vi "new FGGA Serial Data Server & Recordingv4.3_test.vi"(0 "VISA resource name out":refnum<visa-resource-name>, 11 "error IO":errorcluster) -> ()   [LabVIEW 2014]
uses:
  <vilib>/Platform/TimedLoop/XDataNode/timing_clust.ctl
  <vilib>/Platform/TimedLoop/XDataNode/nitl_modes.ctl
  <vilib>/Platform/TimedLoop/XDataNode/wakeup.ctl
  C:/Program Files (x86)/National Instruments/LabVIEW 2014/examples/Data Communication/Network Streams/Simple Network Streams/support/Network Stream Command.ctl
  <vilib>/Utility/error.llb/whitespace.ctl
  <vilib>/Instr/_visa.llb/VISA Flush IO Buffer Mask.ctl
  <vilib>/Instr/_visa.llb/VISA Configure Serial Port (Instr).vi
  <vilib>/Utility/tcp.llb/UDP Multicast Write-Only Open.vi
  <vilib>/platform/TimedLoop/XDataNode/XDataNode.xnode
  <vilib>/Platform/TimedLoop/XDataNode/XDNodeRunTimeDep.lvlib
panel:
  out "Waveform Chart":u32(graph)
  out "Max time diff":u32
  out "ASCII_file_out":string
  out "Unix time":u32
  out "FGGA Pump":bool
  out "Flight Number":string
  out "Stop File Write":bool
  out "Default file name":string
  out "MFC":dbl[](array[numeric])
  out "FGGA restart":bool
  out "V4":bool
  out "V3":bool
  out "V2":bool
  out "V1":bool
  out "error out 2":errorcluster
  out "error out":errorcluster
  in  "MFC_1 SLPM set value":dbl
  out "Value Read":string
  out "status":bool
  in  "VISA resource name":refnum<visa-resource-name>="ASRL3::INSTR"
  in  "timeout (10sec) 2":u32=3000
  in  "Clear Display\nErrors":bool
  out "Data Processing":bool
  out "TCP Binary Packet":string
  out "UDP Time Stamp Offset":i32=1
  out "Data String":string
  out "UDP_ACSII_Out":string
  out "Serial error out":errorcluster
  out "SEPTIC TCP Error Out":errorcluster
  out "TCP packet\nSend To SEPTIC":bool
  out "FISH TCP Error Out":errorcluster
  out "TCP packet\nSend To FISH":bool
  out "UDP_Pack_num":u32
  out "UDP_Out Status":bool
  out "UDP_Out_Error Out":errorcluster
  out "Data Array":string[](array[string])
  out "RAW DATA":string
  in  "stop":bool
  out "Number of times \nRead time out":u32
  out "Loop count":i32
  # "Date"
  # "Time"
  # "CH4_wet_ppm"
  # "1"
  # "CO4_wet_ppm_sd"
  # "H2O_ppm"
  # "3"
  # "H2O_ppm_sd"
  # "CO2_wet_ppm"
  # "5"
  # "CO2_wet_ppm_sd"
  # "CH4_dry_ppm"
  # "CH4_dry_ppm_sd"
  # "CO2_dry_ppm"
  # "CO2_dry_ppm_sd"
  # "cell_pressure_torr"
  # "11"
  # "cell_pressure_torr_sd"
  # "13"
  # "cell_temp_degC"
  # "cell_temp_degC_sdev"
  # "ambient(bench)_temp_degC"
  # "15"
  # "ambient(bench)_temp_dedgC_sd"
  # "17"
  # "RDA_us"
  # "RDA_us_sd"
  # "RDB_us"
  # "19"
  # "RDB_us_sd"
  # "Fitflag"
  # "21"
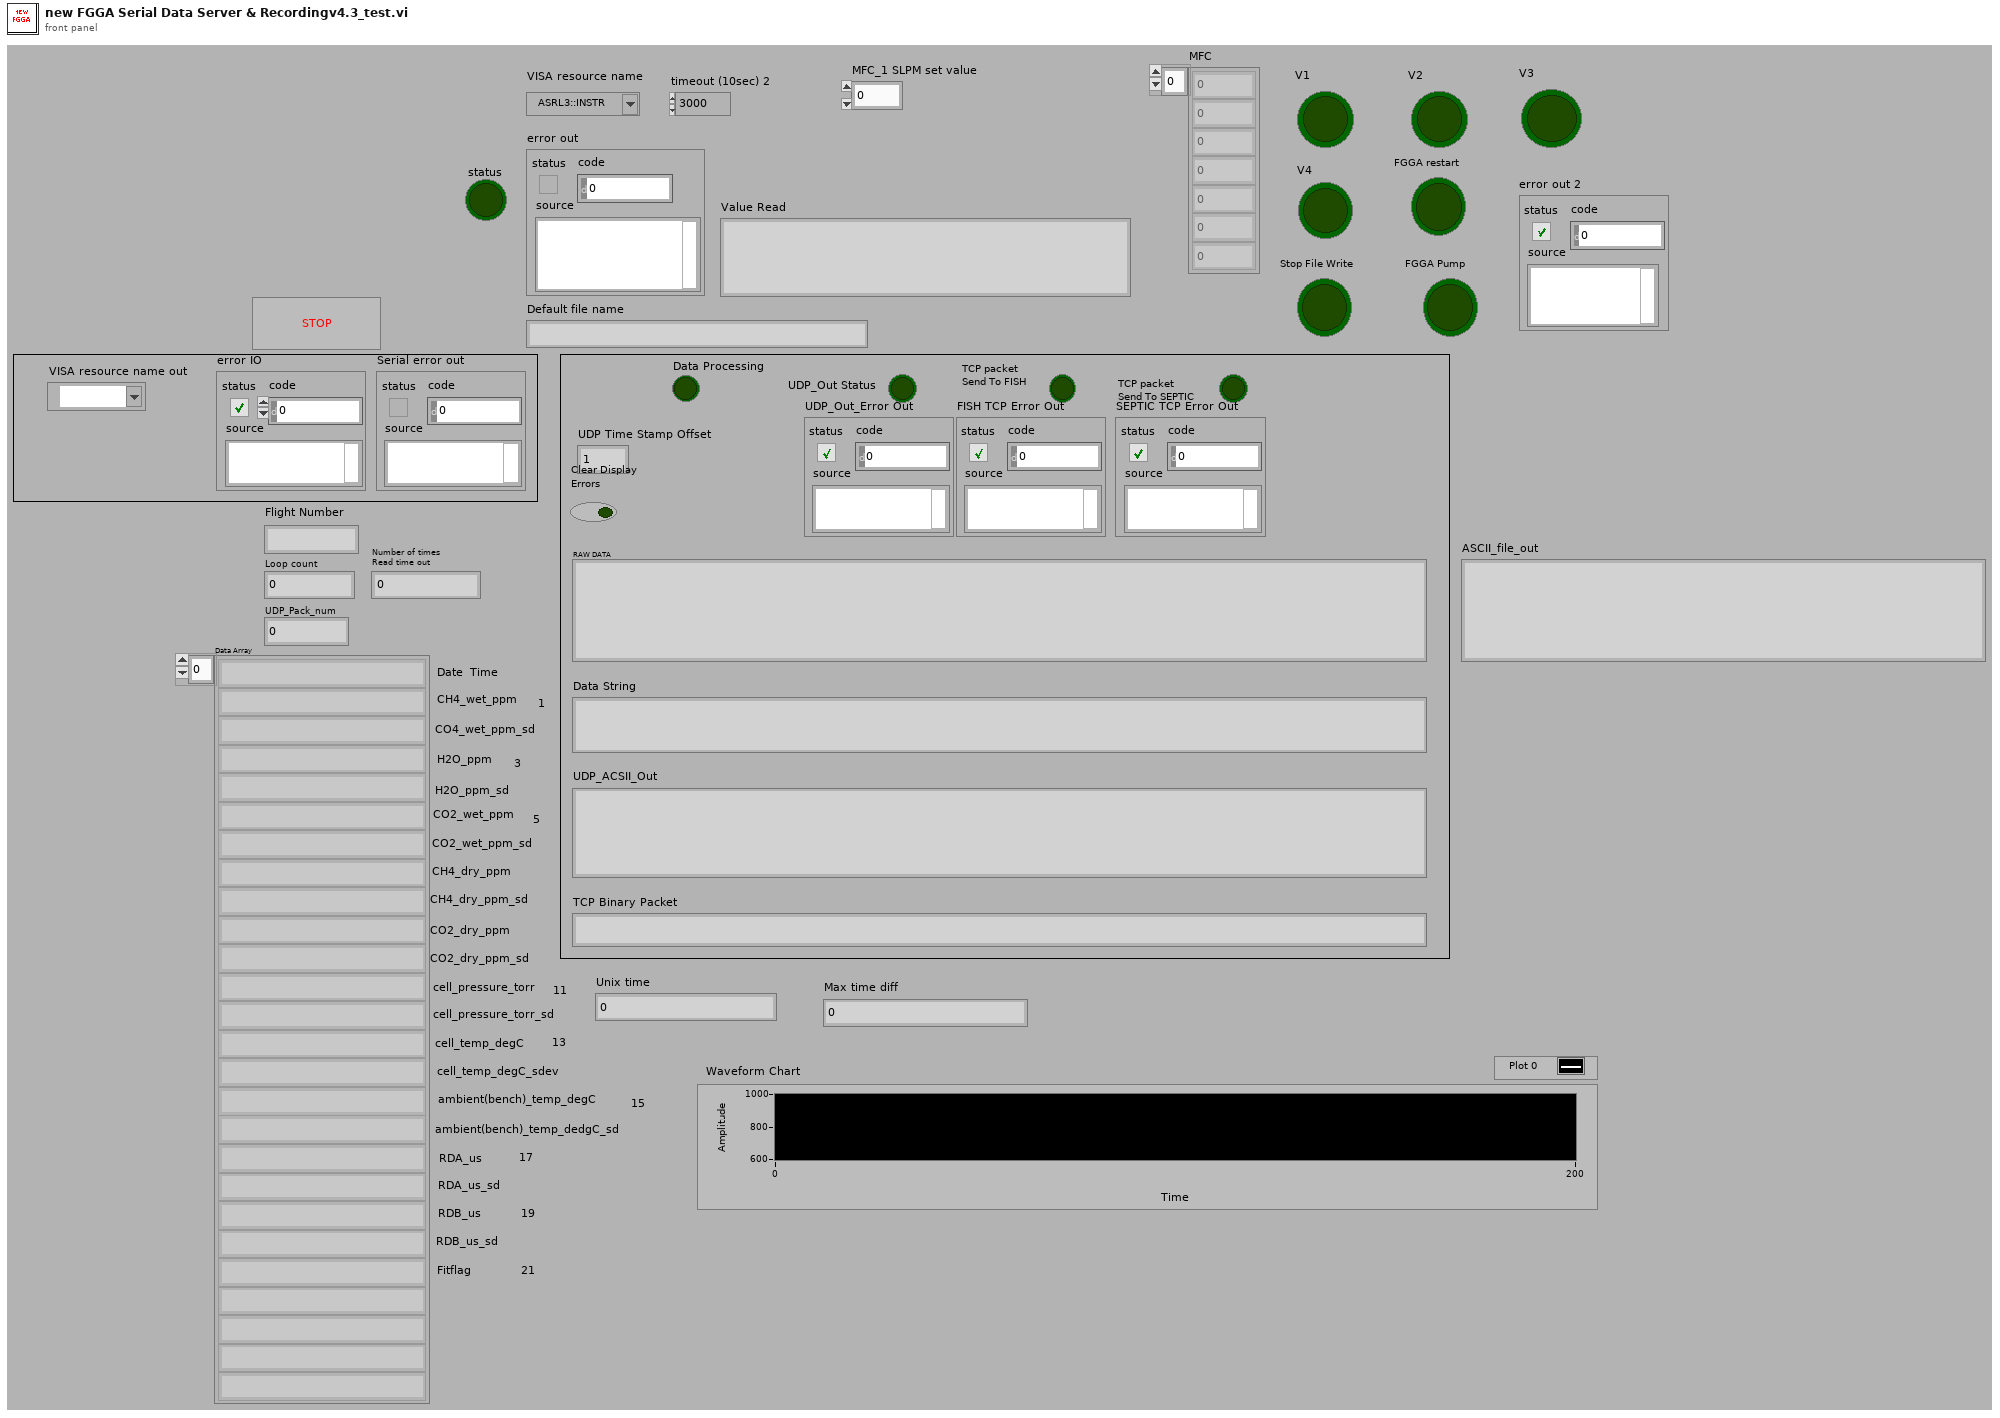
[diagram p1: front panel]
types:
  T1 = typedef "XDNodeRunTimeDep.lvlib/timing_clust.ctl" = cluster{"Expected End [f-1]":u64, "Actual End [f-1]":u64, "Finished Late? [f-1]":bool, "Expected End [i-1]":u64, "Actual End [i-1]":u64, "Finished Late? [i-1]":bool, "Expected Start [i]":u64, "Actual Start [i]":u64, "Expected Start [f]":u64, "Actual Start [f]":u64, "Source Name":string, "Structure Name":string, "Period":i64, "Deadline":i64, "Offset":i64, "Start":i64, "Priority":i32, "Timeout":i32, "Mode":T2, "Wakeup Reason":T3, "Error":errorcluster, "Source Type":string, "Secondary Source Type":string, "Global End Time":u64, "Global Start Time":u64, "Frame Duration":u64, "Iteration Duration":u64, "Assigned CPU":i32, "I/O Scan Engine Mode":u32}
  T2 = typedef "XDNodeRunTimeDep.lvlib/nitl_modes.ctl" = enum32{"No Change", "Process missed periods, maintain original phase", "Discard missed periods, maintain original phase", "Process missed periods, ignore original phase", "Discard missed periods, ignore original phase"}
  T3 = typedef "XDNodeRunTimeDep.lvlib/wakeup.ctl" = enum32{"Normal", "Aborted", "Asynchronous wakeup", "Timing source error", "Timed loop error", "Timeout"}
  T4 = enum16{"open", "replace", "create", "open or create", "replace or create", "replace or create with confirmation"}
  T5 = typedef "Network Stream Command.ctl" = cluster{"Message":string, "Message Data":variant}
  T6 = typedef "whitespace.ctl" = u16
  T7 = typedef "VISA Flush IO Buffer Mask.ctl" = u16
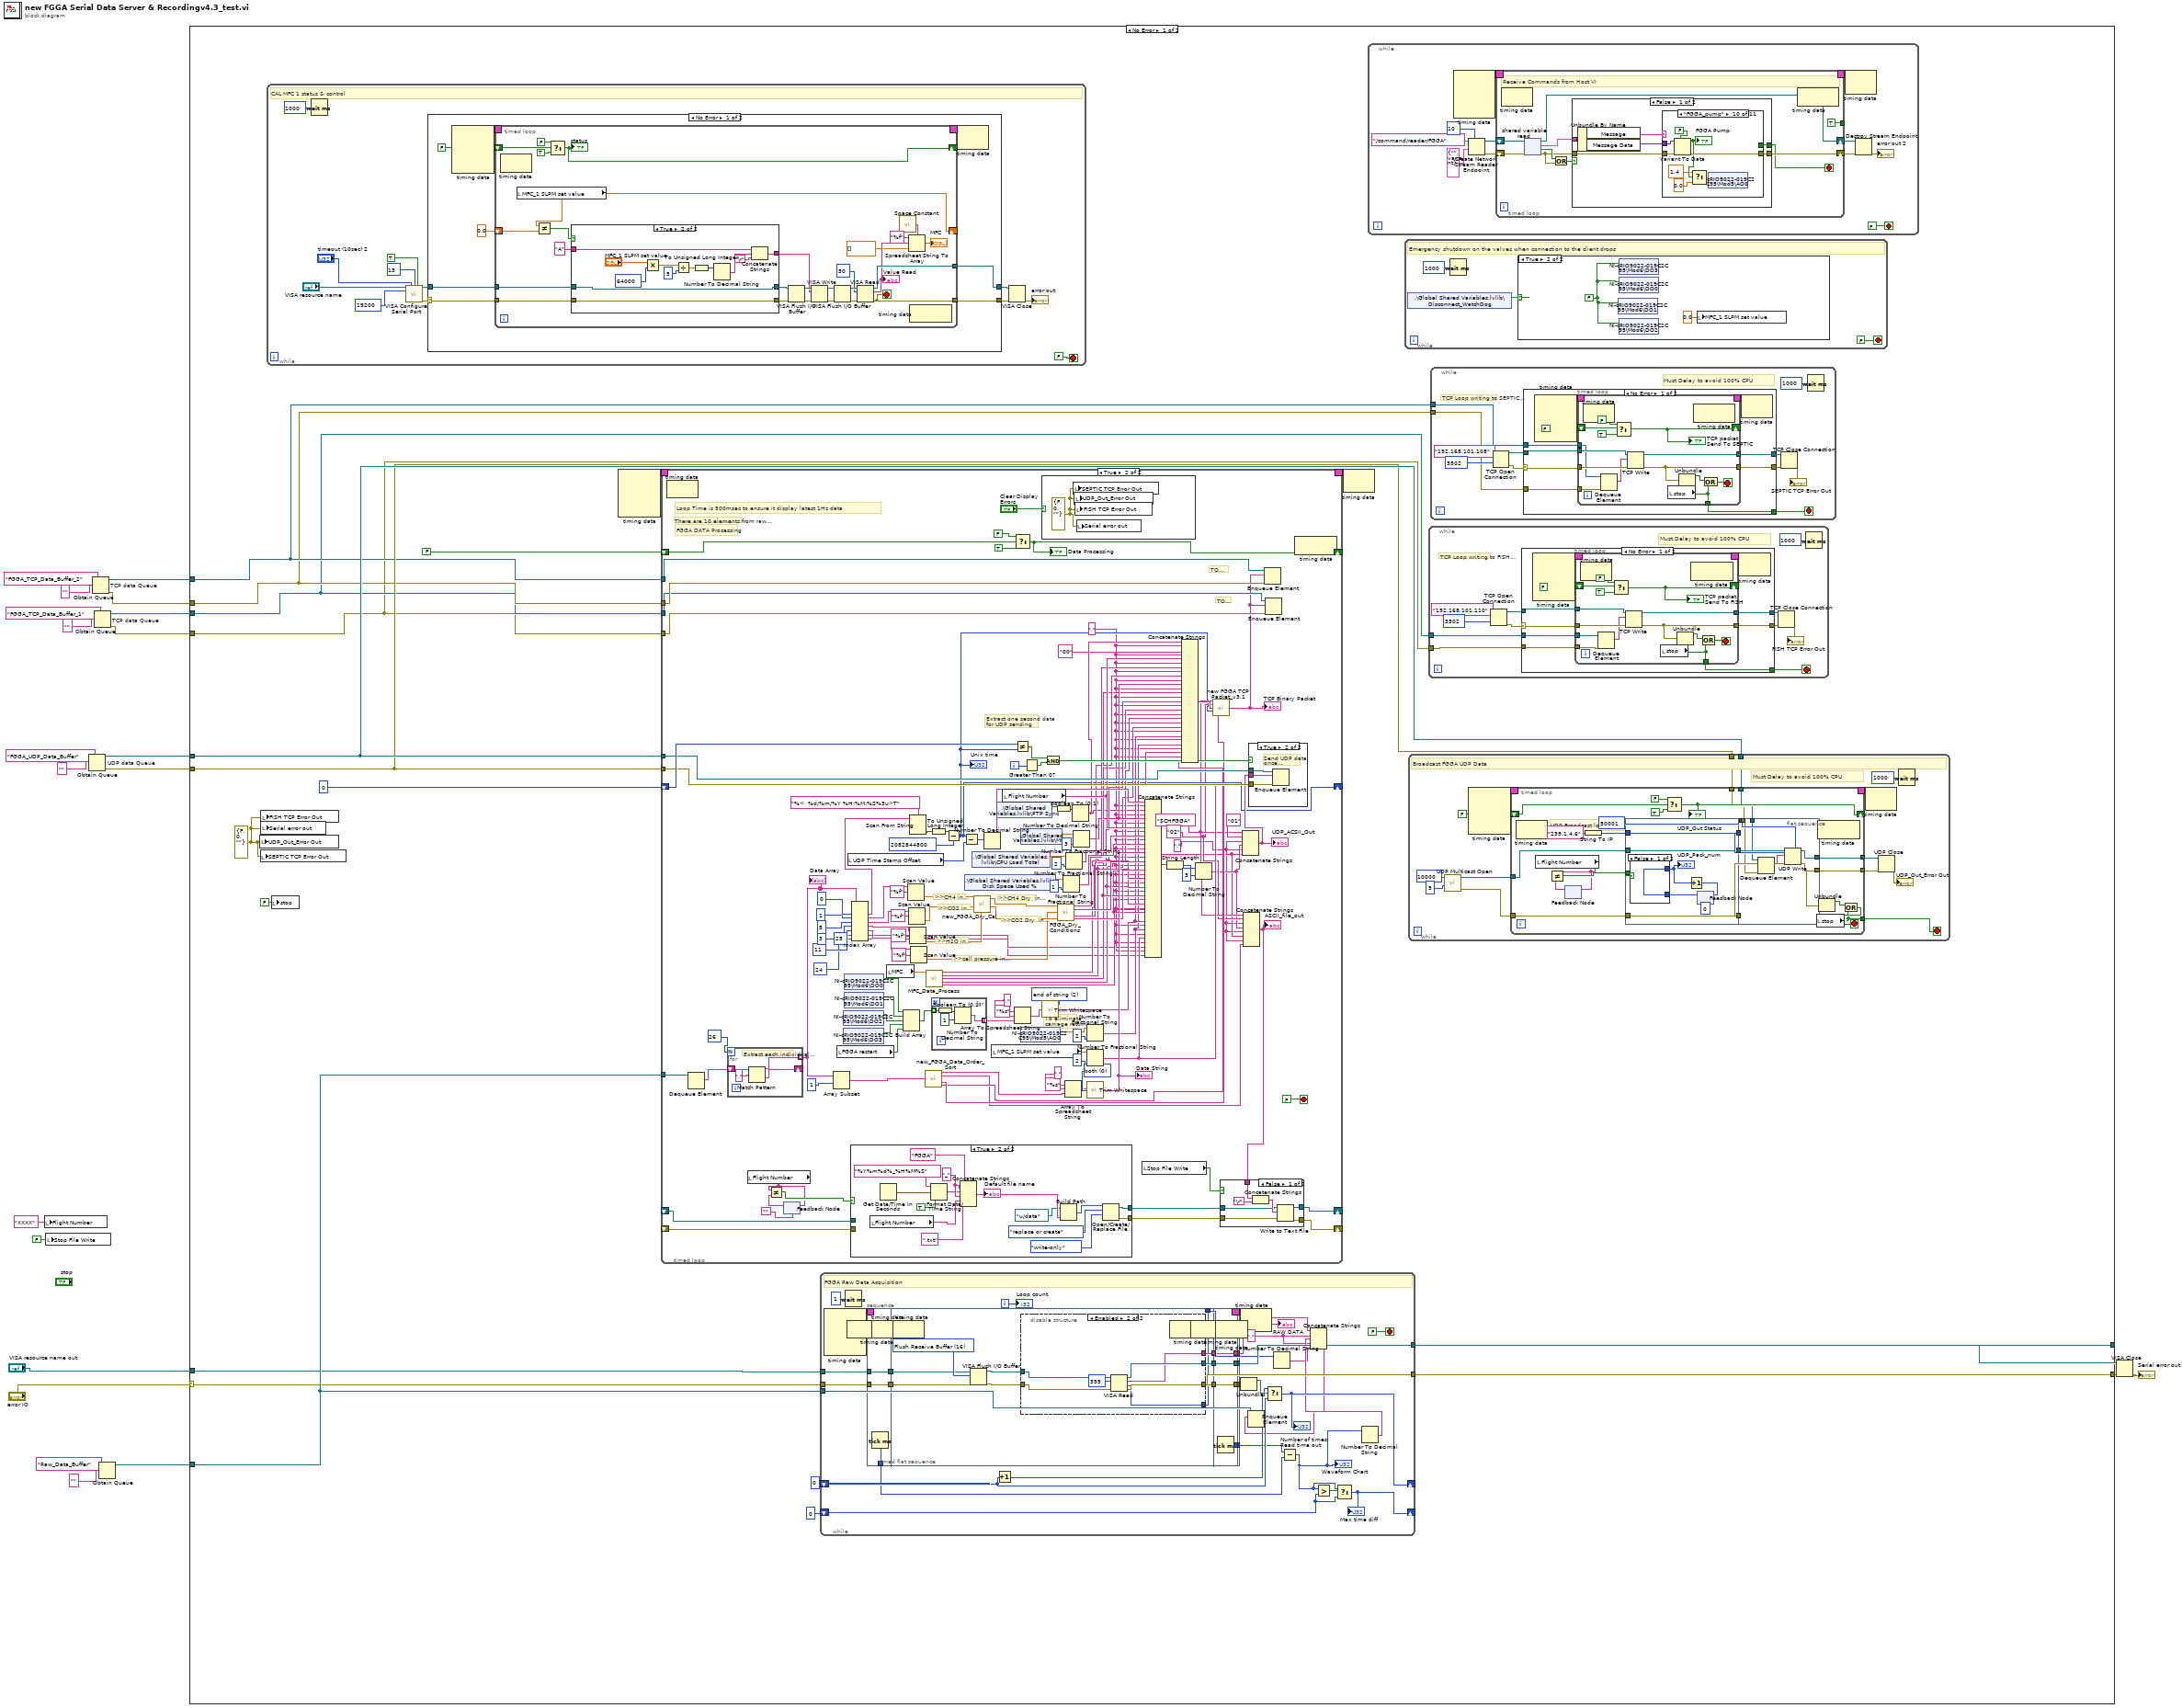
[diagram p0: block diagram]
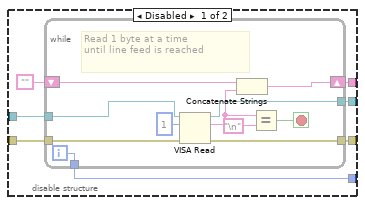
[diagram p2: hidden frame]
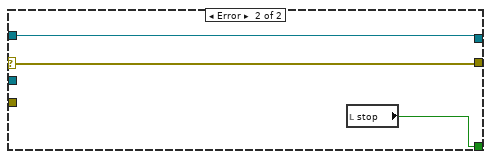
[diagram p3: hidden frame]
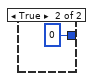
[diagram p4: hidden frame]
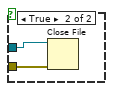
[diagram p6: hidden frame]
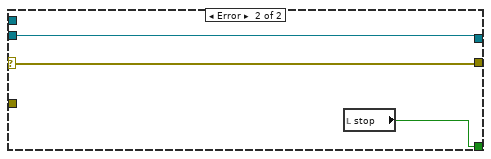
[diagram p9: hidden frame]
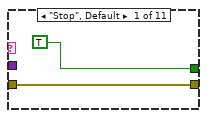
[diagram p11: hidden frame]
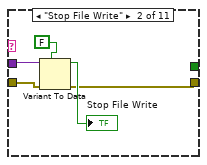
[diagram p12: hidden frame]
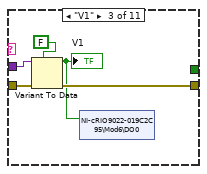
[diagram p13: hidden frame]
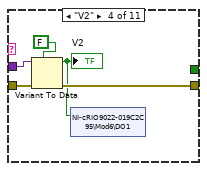
[diagram p14: hidden frame]
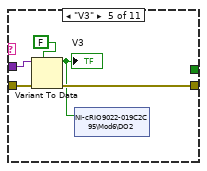
[diagram p15: hidden frame]
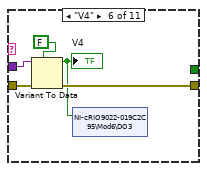
[diagram p16: hidden frame]
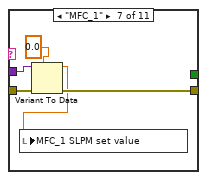
[diagram p17: hidden frame]
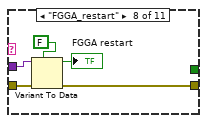
[diagram p18: hidden frame]
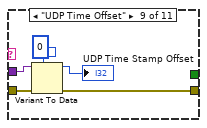
[diagram p19: hidden frame]
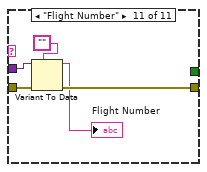
[diagram p20: hidden frame]
diagram:
  n1 = local write "Flight Number"("XXXX" ("Flight Number")) -> ()
  n2 = local write "Stop File Write"(FALSE ("Stop File Write")) -> ()
  n3 = Obtain Queue "UDP data Queue"(name (unnamed)="FGGA_UDP_Data_Buffer", element data type="") -> (queue out=w14:refnum<queue>, error out=w13:errorcluster)  [unwired: 3 in, 1 out]
  n4 = Obtain Queue "TCP data Queue"(name (unnamed)="FGGA_TCP_Data_Buffer_2", element data type="") -> (queue out=w8:refnum<queue>, error out=w7:errorcluster)  [unwired: 3 in, 1 out]
  n5 = Obtain Queue "TCP data Queue"(name (unnamed)="FGGA_TCP_Data_Buffer_1", element data type="") -> (queue out=w6:refnum<queue>, error out=w5:errorcluster)  [unwired: 3 in, 1 out]
  n6 = Obtain Queue(name (unnamed)="Raw_Data_Buffer", element data type="") -> (queue out=w20:refnum<queue>)  [unwired: 3 in, 2 out]
  n7 = case shown="No Error" "error IO" {
    selector: "error IO" -> [w28 w608]
    tunnel: "VISA resource name out" -> [w29 w609]
    tunnel: [w40 w609] -> w17
    tunnel: [w41 w608] -> w18
    tunnel: w20 -> [w39 _]
    tunnel: w14 -> [w37 _]
    tunnel: w13 -> [w36 _]
    tunnel: w8 -> [w35 _]
    tunnel: w7 -> [w34 _]
    tunnel: w6 -> [w33 _]
    tunnel: w5 -> [w32 _]
    frame No Error {
      w25 = errorcluster {"status"=FALSE, "code"=0, "source"=""} ("UDP Error Out")
      n8 = local write "UDP_Out_Error Out"(w25) -> ()
      n9 = local write "SEPTIC TCP Error Out"(w25) -> ()
      n10 = local write "FISH TCP Error Out"(w25) -> ()
      n11 = local write "Serial error out"(w25) -> ()
      n12 = while {
        stop <- FALSE stop-if-true
        # "CAL MFC 1 status & control"
        n13 = Wait (ms)(milliseconds to wait=u32 1000) -> ()  [unwired: 1 out]
        n14 = call-poly "VISA Configure Serial Port"("VISA resource name"="VISA resource name", "timeout (10sec)"="timeout (10sec) 2", "termination char\n(0xA = '\\n' = LF)"=u8 13 ("termination char\n(0xA = '\\n' = LF)"), "Enable Termination\nChar (T)"=TRUE ("Enable Termination\nChar (T)"), "baud rate (9600)"=u32 19200) -> ("VISA resource name out"=w549:refnum<visa-resource-name>, "error out"=w545:errorcluster)  [unwired: 9 in]
        n15 = case shown="No Error" w545 {
          selector: w545 -> [w556 w606]
          tunnel: w549 -> [w557 w607]
          tunnel: [w555 w607] -> w548
          tunnel: [w554 w606] -> w547
          frame No Error {
            n16 = node-c288() -> (w552:T1)  [unwired: 4 in]
            n17 = timed-loop {
              tunnel: w557 -> [w580]
              tunnel: w556 -> [w578]
              tunnel: [w571] -> w555
              tunnel: [w566] -> w554
              shift-right: [w567] -> _
              shift-left: FALSE -> [w570]
              timing: w552 -> [_]
              timing-out: [_] -> w551
              shift-right: [w558] -> _
              shift-left: 0.0 -> [w560]
              stop <- w566 stop-if-true
              n18 = node-c288() -> ()  [unwired: 1 in, 1 out]
              n19 = local read "MFC_1 SLPM set value"() -> (w558:dbl)
              n20 = Not Equal?(x=w558, y=w560) -> (x != y?=w559:bool)
              n21 = Select(t=FALSE, s=w570, f=TRUE) -> (s? t:f=w567:bool)
              "status" <- w567
              n22 = case shown="True" w559 {
                tunnel: w580 -> [w588 w603]
                tunnel: [w588 w603] -> w579
                tunnel: w578 -> [w587 w602]
                tunnel: [w587 w602] -> w577
                tunnel: "A" -> [w591 w595]
                tunnel: [w589 w592] -> w575
                frame False {
                  n23 = Concatenate Strings(w591, "\r") -> (w589:string)
                }
                frame True {
                  n24 = Multiply(x="MFC_1 SLPM set value", y=u32 64000) -> (x*y=w599:dbl)
                  n25 = Divide(x=w599, y=u32 5) -> (x/y=w597:dbl)
                  n26 = To Unsigned Long Integer(number=w597) -> (unsigned 32bit integer=w596:u32)
                  n27 = Number To Decimal String(number=w596) -> (decimal integer string=w594:string)  [unwired: 1 in]
                  n28 = Concatenate Strings(w595, w594, "\r") -> (w592:string)
                }
              }
              n29 = VISA Flush I/O Buffer(VISA resource name=w579, error in (no error)=w577) -> (VISA resource name out=w582:refnum<visa-resource-name>, error out=w581:errorcluster)  [unwired: 1 in]
              n30 = VISA Write(VISA resource name=w582, write buffer=w575, error in (no error)=w581) -> (VISA resource name out=w574:refnum<visa-resource-name>, error out=w573:errorcluster)  [unwired: 1 out]
              n31 = VISA Flush I/O Buffer(VISA resource name=w574, error in (no error)=w573) -> (VISA resource name out=w584:refnum<visa-resource-name>, error out=w583:errorcluster)  [unwired: 1 in]
              n32 = VISA Read(VISA resource name=w584, byte count=u32 50, error in (no error)=w583) -> (VISA resource name out=w571:refnum<visa-resource-name>, read buffer=w565:string, error out=w566:errorcluster)  [unwired: 1 out]
              "Value Read" <- w565
              n33 = call <vilib>:"Space Constant.vi"() -> ("String"=w564:string)
              n34 = Spreadsheet String To Array(delimiter (Tab)=w564, format string="%f", spreadsheet string=w565, array type (2D Dbl)=dbl[] []) -> (array=→"MFC":dbl[])
              n35 = node-c288() -> ()  [unwired: 1 in, 1 out]
            }
            n36 = node-c288(w551) -> ()  [unwired: 1 out]
          }
          frame Error {
          }
        }
        n37 = VISA Close(VISA resource name=w548, error in (no error)=w547) -> (error out=→"error out":errorcluster)
      }
      n38 = local write "stop"(FALSE ("stop")) -> ()
      n39 = node-c288() -> (w27:T1)  [unwired: 4 in]
      n40 = timed-loop {
        timing: w27 -> [_]
        timing-out: [_] -> w26
        tunnel: w39 -> [w360]
        tunnel: w37 -> [w328]
        tunnel: w36 -> [w327]
        shift-right: [w255] -> _
        shift-left: u32 0 -> [w331]
        tunnel: w35 -> [w326]
        tunnel: w34 -> [w325]
        tunnel: w33 -> [w324]
        tunnel: w32 -> [w323]
        shift-right: [w319] -> _
        shift-left: FALSE -> [w322]
        shift-right: [w308] -> _
        shift-left: _ -> [w300]
        shift-right: [w298] -> _
        shift-left: _ -> [w299]
        i -> [w330]
        stop <- FALSE stop-if-true
        w272 = T6 2 items=["both", "start of string", "end of string"] ("location (both)")
        w233 = ","
        w349 = T6 0 items=["both", "start of string", "end of string"] ("location (both)")
        w237 = ","
        w241 = "02"
        w242 = "$CHFGGA"
        # "To eliminate\ncarriage return"
        # ">>cell pressure in torr>>"
        # "There are 10 elements from raw packet"
        # "TO SEPTIC"
        # "TO FISH"
        # "Extract one second data\nfor UDP sending"
        # ">>CO2 Dry  in ppm>>"
        # ">>CH4 Dry  in ppb>>"
        # ">>H2O in ppm>>"
        # ">>CO2 in ppm>>"
        # ">>CH4 in ppm>>"
        # "Loop Time is 500msec to ensure it display latest 1Hz data"
        # "FGGA DATA Processing"
        n41 = node-c288() -> ()  [unwired: 1 in, 1 out]
        n42 = Dequeue Element(queue=w360) -> (element=w318:string)  [unwired: 2 in, 3 out]
        n43 = for {
          N: 26 -> [_]
          shift-right: [w397] -> _
          shift-left: w318 -> [w395]
          tunnel: [w396] -> w354 mode=indexing
          # "Extract each individual param"
          n44 = Match Pattern(string=w395, regular expression=",") -> (before substring=w396:string, after substring=w397:string)  [unwired: 1 in, 2 out]
        }
        "Data Array" <- w354
        n45 = local read "Flight Number"() -> (w297:string)
        n46 = feedback #1("" ("Flight Number")) -> (w305:string)
        n47 = Not Equal?(x=w297, y=w305) -> (x != y?=w303:bool)
        n48 = feedback-in #1(w297) -> ()
        n49 = Array Subset(array=w354, index=1) -> (w247:string[])  [unwired: 1 in]
        n50 = local read "FGGA restart"() -> (w282:bool)
        n51 = shared-variable "NI-cRIO9022-019C2C95\\Mod6\\DO2"() -> (w288:bool)  [unwired: 1 in, 1 out]
        n52 = shared-variable "NI-cRIO9022-019C2C95\\Mod6\\DO3"() -> (w287:bool)  [unwired: 1 in, 1 out]
        n53 = shared-variable "NI-cRIO9022-019C2C95\\Mod6\\DO0"() -> (w290:bool)  [unwired: 1 in, 1 out]
        n54 = shared-variable "NI-cRIO9022-019C2C95\\Mod6\\DO1"() -> (w289:bool)  [unwired: 1 in, 1 out]
        n55 = local read "UDP Time Stamp Offset"() -> (w271:i32)
        n56 = case shown="True" w303 {
          tunnel: [w366 w368] -> w302
          tunnel: [w365 w367] -> w301
          tunnel: w300 -> [w366 _]
          tunnel: w299 -> [w365 _]
          frame False {
          }
          frame True {
            w374 = "_" ("string")
            n57 = local read "Flight Number"() -> (w381:string)
            n58 = Get Date/Time In Seconds() -> (seconds since 1Jan1904=w369:timestamp)
            n59 = Format Date/Time String(time format string (%c)="%Y%m%d%_%H%M%S", seconds (now)=w369, UTC format=TRUE) -> (date/time string=w371:string)
            n60 = Concatenate Strings("FGGA" ("string"), w374, w371, w374, w381, ".txt" ("string")) -> (w376:string)
            "Default file name" <- w376
            n61 = Build Path(base path=path "u:/data", name or relative path=w376) -> (appended path=w380:path)
            n62 = Open/Create/Replace File(file path (use dialog)=w380, operation (0:open)=T4."replace or create", access (0:read/write)=enum16{"read/write", "read-only", "write-only"}."write-only") -> (refnum out=w368:refnum<file>, error out=w367:errorcluster)  [unwired: 3 in, 1 out]
          }
        }
        n63 = Index Array(array=w354, index #1=0 ("index"), index #2=1 ("index"), index #3=5 ("index"), index #4=3 ("index"), index #5=11 ("index"), index #6=24 ("index"), index #7=25 ("index")) -> (element #1=w249:string, element #2=w254:string, element #3=w253:string, element #4=w252:string, element #5=w251:string, element #6=w234:string, element #7=w231:string)
        n64 = local read "MFC"() -> (w309:dbl[])
        n65 = Build Array(w290, w289, w288, w287, w282) -> (w286:bool[])
        n66 = Scan Value(string=w254, format string="%f") -> (value=w340:dbl)  [unwired: 1 in, 1 out]
        n67 = Scan Value(string=w253, format string="%f") -> (value=w339:dbl)  [unwired: 1 in, 1 out]
        n68 = Scan From String(format string="%<  %d/%m/%Y %H:%M:%S%3u>T", input string=w249) -> (output 1=w336:timestamp)  [unwired: 3 in, 3 out]
        n69 = Scan Value(string=w252, format string="%f") -> (value=w310:dbl)  [unwired: 1 in, 1 out]
        n70 = Scan Value(string=w251, format string="%f") -> (value=w311:dbl)  [unwired: 1 in, 1 out]
        n71 = call "new_FGGA_Data_Order_Sort.vi"("Data In"=w247) -> ("UDP Data Out"=w246:string[], "ASCII Ambient(bench)_temp"=w236:string, "TCP Data Out"=w245:string[], "TCP Ambient(bench)_temp"=w244:string)  [unwired: 11 in]
        n72 = call "MFC_Data_Process.vi"("MFC"=w309) -> ("MFC Absolute Pressure"=w266:string, "MFC Temperature"=w265:string, "MFC Volumetric Flow"=w264:string, "MFC Mass Flow"=w263:string, "MFC Set Point"=w262:string)  [unwired: 10 in]
        n73 = To Unsigned Long Integer(number=w336) -> (unsigned 32bit integer=w337:u32)
        n74 = for {
          tunnel: w286 -> [w363] mode=indexing
          tunnel: [w362] -> w283 mode=indexing
          n75 = Boolean To (0,1)(Boolean=w363) -> (0, 1=w364:i16)
          n76 = Number To Decimal String(number=w364, width (-)=i16 1) -> (decimal integer string=w362:string)
        }
        n77 = Subtract(x=w337, y=u32 2082844800) -> (x-y=w255:u32)
        "Unix time" <- w255
        n78 = Subtract(x=w255, y=w271) -> (x-y=w334:u32)
        n79 = shared-variable ".\\Global Shared Variables.lvlib\\Disk Space Used %"() -> (w275:dbl)  [unwired: 1 in, 1 out]
        n80 = shared-variable ".\\Global Shared Variables.lvlib\\CPU Load Total"() -> (w296:dbl)  [unwired: 1 in, 1 out]
        n81 = call "new_FGGA_Dry_Cal.vi"("H2O"=w310, "CO2_Wet"=w339, "CH4_Wet"=w340) -> ("CO2_Dry"=w313:dbl, "CH4_Dry"=w315:dbl)  [unwired: 7 in]
        n82 = Number To Decimal String(number=w334) -> (decimal integer string=w335:string)  [unwired: 1 in]
        n83 = local read "MFC_1 SLPM set value"() -> (w278:dbl)
        n84 = shared-variable ".\\Global Shared Variables.lvlib\\PTP Sync"() -> (w291:bool)  [unwired: 1 in, 1 out]
        n85 = local read "Flight Number"() -> (w270:string)
        n86 = Array To Spreadsheet String(delimiter (Tab)=",", array=w283, 3:"%s" ("format string")) -> (spreadsheet string=w273:string)
        n87 = Select(t=FALSE, s=w322, f=TRUE) -> (s? t:f=w319:bool)
        "Data Processing" <- w319
        n88 = Not Equal?(x=w331, y=w255) -> (x != y?=w332:bool)
        n89 = shared-variable ".\\Global Shared Variables.lvlib\\MFM"() -> (w294:dbl)  [unwired: 1 in, 1 out]
        n90 = shared-variable "NI-cRIO9022-019C2C95\\Mod5\\AO0"() -> (w280:dbl)  [unwired: 1 in, 1 out]
        n91 = Greater Than 0?(x=w330) -> (x > 0?=w333:bool)
        n92 = case shown="True" "Clear Display\nErrors" {
          frame False {
          }
          frame True {
            w391 = errorcluster {"status"=FALSE, "code"=0, "source"=""} ("UDP Error Out")
            n93 = local write "SEPTIC TCP Error Out"(w391) -> ()
            n94 = local write "UDP_Out_Error Out"(w391) -> ()
            n95 = local write "FISH TCP Error Out"(w391) -> ()
            n96 = local write "Serial error out"(w391) -> ()
          }
        }
        n97 = call <vilib>:"Trim Whitespace.vi"("string"=w273, "location (both)"=w272) -> ("trimmed string"=w261:string)
        n98 = Compound Arithmetic op=AND(w332, w333) -> (w329:bool)
        n99 = Boolean To (0,1)(Boolean=w291) -> (0, 1=w292:i16)
        n100 = call "FGGA_Dry_Conditions.vi"("CH4_Dry"=w315, "Pressure"=w311, "CO2_Dry"=w313) -> ("CH4_Dry_TCP"=w269:string, "CH4_Dry_UDP"=w317:string, "CO2_Dry_TCP"=w268:string, "CO2_Dry_UDP"=w316:string)  [unwired: 9 in]
        n101 = Number To Fractional String(number=w275, precision (6)=i16 1) -> (F-format string=w274:string)  [unwired: 2 in]
        n102 = Array To Spreadsheet String(delimiter (Tab)=",", array=w246, 3:"%s" ("format string")) -> (spreadsheet string=w348:string)
        n103 = Number To Fractional String(number=w296, precision (6)=i16 2) -> (F-format string=w277:string)  [unwired: 2 in]
        n104 = Number To Decimal String(number=w292) -> (decimal integer string=w257:string)  [unwired: 1 in]
        n105 = Number To Fractional String(number=w294, precision (6)=i16 3) -> (F-format string=w267:string)  [unwired: 2 in]
        n106 = Number To Fractional String(number=w280, precision (6)=i16 2) -> (F-format string=w260:string)  [unwired: 2 in]
        n107 = Number To Fractional String(number=w278, precision (6)=i16 2) -> (F-format string=w259:string)  [unwired: 2 in]
        n108 = call <vilib>:"Trim Whitespace.vi"("string"=w348, "location (both)"=w349) -> ("trimmed string"=w347:string)
        "Data String" <- w347
        n109 = local read "Stop File Write"() -> (w306:bool)
        n110 = Concatenate Strings(w335, w233, w257, w233, w267, w233, w270, w233, w277, w233, w274, w233, w347, w233, w317, w233, w316, w233, w266, w233, w265, w233, w264, w233, w263, w233, w262, w233, w261, w233, w260, w233, w259, w233, w234, w233, w231) -> (w239:string)
        n111 = String Length(string=w239) -> (length=w357:i32)
        n112 = Concatenate Strings(w257, w233, "00", w233, w270, w233, w269, w233, w268, w233, w267, w233, w266, w233, w265, w233, w264, w233, w263, w233, w262, w233, w261, w233, w260, w233, w259, w233, w244) -> (w258:string)
        n113 = Number To Decimal String(number=w357, width (-)=i16 3) -> (decimal integer string=w240:string)
        n114 = call "new FGGA TCP Packet_v3.1.vi"("ID"=w242, "Version"=w241, "TCP Packet In"=w258, "utc_time"=w255, "Data Array"=w245) -> ("TCP Binary Packet"=w248:string)  [unwired: 10 in]
        "TCP Binary Packet" <- w248
        n115 = Concatenate Strings(w242, "01", w237, w240, w237, w239) -> (w307:string)
        "UDP_ACSII_Out" <- w307
        n116 = Concatenate Strings(w242, w241, w237, w240, w237, w239, w237, w236) -> (w238:string)
        "ASCII_file_out" <- w238
        n117 = case shown="False" w306 {
          tunnel: w238 -> [w388 _]
          tunnel: [w385 _] -> w308
          tunnel: w302 -> [w384 w390]
          tunnel: w301 -> [w383 w389]
          tunnel: [w382 _] -> w298
          frame False {
            n118 = Concatenate Strings(w388, "\r") -> (w386:string)
            n119 = Write to Text File(file (use dialog)=w384, text=w386, error in=w383) -> (refnum out=w385:refnum<file>, error out=w382:errorcluster)  [unwired: 2 out]
          }
          frame True {
            n120 = Close File(refnum=w390, error in=w389) -> ()  [unwired: 2 out]
          }
        }
        n121 = case shown="True" w329 {
          tunnel: w307 -> [_ w394]
          tunnel: w328 -> [_ w393]
          tunnel: w327 -> [_ w392]
          frame False {
          }
          frame True {
            # "Send UDP data once\na second"
            n122 = Enqueue Element(queue=w393, element=w394, error in (no error)=w392) -> ()  [unwired: 1 in, 3 out]
          }
        }
        n123 = Enqueue Element(queue=w326, element=w248, error in (no error)=w325) -> ()  [unwired: 1 in, 3 out]
        n124 = Enqueue Element(queue=w324, element=w248, error in (no error)=w323) -> ()  [unwired: 1 in, 3 out]
        n125 = node-c288() -> ()  [unwired: 1 in, 1 out]
      }
      n126 = while {
        tunnel: w29 -> [w57]
        tunnel: w28 -> [w56]
        tunnel: [w67] -> w41
        shift-right: [w63] -> _
        shift-left: u32 0 -> [w64]
        tunnel: [w66] -> w40
        tunnel: w39 -> [w61]
        shift-right: [w51] -> _
        shift-left: u32 0 -> [w52]
        i -> [w65]
        stop <- FALSE stop-if-true
        w45 = ","
        # "FGGA Raw Data Acquisition"
        n127 = node-c288() -> (w43:T1)  [unwired: 4 in]
        n128 = Wait (ms)(milliseconds to wait=u32 1) -> ()  [unwired: 1 out]
        n129 = timed-sequence {
          timing: w43 -> [_]
          timing-out: [_] -> w42
          tunnel: w57 -> [w80]
          tunnel: w56 -> [w79]
          tunnel: [w78] -> w54
          tunnel: [w75] -> w46
          tunnel: [w73] -> w67
          tunnel: [w71] -> w66
          tunnel: [w69] -> w49
          tunnel: [w68] -> w55
          n130 = timed-flat-sequence {
            tunnel: w79 -> [w82]
            tunnel: w80 -> [w83]
            tunnel: [w83] -> w77
            tunnel: [w82] -> w76
            tunnel: [w81] -> w78
            tunnel: w77 -> [w88]
            tunnel: w76 -> [w87]
            tunnel: [w94] -> w74
            tunnel: [w93] -> w72
            tunnel: [w92] -> w70
            tunnel: [w86] -> w75
            tunnel: [w123] -> w69
            tunnel: [w124] -> w71
            tunnel: [w125] -> w73
            tunnel: w74 -> [w125]
            tunnel: w72 -> [w124]
            tunnel: w70 -> [w123]
            tunnel: [w122] -> w68
            frame #0 {
              n131 = node-c288() -> ()  [unwired: 1 in, 1 out]
              n132 = node-c288() -> ()  [unwired: 1 in, 1 out]
              n133 = Tick Count (ms)() -> (millisecond timer value=w81:u32)
            }
            frame #1 {
              w89 = T7 16 items=["Flush Receive Buffer"=16, "Write Transmit Buffer to Device"=32, "Flush Receive Buffer (No I/O)"=64, "Flush Transmit Buffer"=128] ("Mask")
              n134 = node-c288() -> ()  [unwired: 1 in, 1 out]
              n135 = VISA Flush I/O Buffer(VISA resource name=w88, mask (16)=w89, error in (no error)=w87) -> (VISA resource name out=w90:refnum<visa-resource-name>, error out=w91:errorcluster)
              n136 = disable-structure shown="Enabled" {
                disable-tunnel: [w103 w119] -> w94
                disable-tunnel: [w102 w118] -> w93
                disable-tunnel: [w101 w117] -> w92
                disable-tunnel: w91 -> [w100 w120]
                disable-tunnel: w90 -> [w99 w121]
                disable-tunnel: [w97 w115] -> w86
                frame Disabled {
                  n137 = while {
                    tunnel: [w114] -> w102
                    tunnel: [w113] -> w103
                    tunnel: w99 -> [w112]
                    tunnel: w100 -> [w111]
                    shift-right: [w109] -> w101
                    shift-left: "" -> [w110]
                    tunnel: [w104] -> w97
                    i -> [w104]
                    stop <- w106 stop-if-true
                    # "Read 1 byte at a time \nuntil line feed is reached"
                    n138 = VISA Read(VISA resource name=w112, byte count=u32 1, error in (no error)=w111) -> (VISA resource name out=w114:refnum<visa-resource-name>, read buffer=w108:string, error out=w113:errorcluster)  [unwired: 1 out]
                    n139 = Concatenate Strings(w110, w108) -> (w109:string)
                    n140 = Equal?(x=w108, y="\n") -> (x = y?=w106:bool)
                  }
                }
                frame Enabled {
                  n141 = VISA Read(VISA resource name=w121, byte count=u32 395, error in (no error)=w120) -> (VISA resource name out=w118:refnum<visa-resource-name>, read buffer=w117:string, return count=w115:u32, error out=w119:errorcluster)
                }
              }
              n142 = node-c288() -> ()  [unwired: 1 in, 1 out]
            }
            frame #2 {
              n143 = node-c288() -> ()  [unwired: 1 in, 1 out]
              n144 = node-c288() -> ()  [unwired: 1 in, 1 out]
              n145 = Tick Count (ms)() -> (millisecond timer value=w122:u32)
            }
          }
        }
        "RAW DATA" <- w49
        n146 = Increment(x=w64) -> (x+1=w62:u32)
        n147 = node-c288(w42) -> ()  [unwired: 1 out]
        n148 = Unbundle(w67) -> ("status"=w60:bool)  [unwired: 2 out]
        n149 = Select(t=w62, s=w60, f=w64) -> (s? t:f=w63:u32)
        "Number of times \nRead time out" <- w63
        n150 = Number To Decimal String(number=w46) -> (decimal integer string=w44:string)  [unwired: 1 in]
        n151 = Subtract(x=w55, y=w54) -> (x-y=w50:u32)
        "Waveform Chart" <- w50
        n152 = Greater?(x=w50, y=w52) -> (0:w53:bool)
        n153 = Select(t=w50, s=w53, f=w52) -> (s? t:f=w51:u32)
        "Max time diff" <- w51
        n154 = Number To Decimal String(number=w50) -> (decimal integer string=w48:string)  [unwired: 1 in]
        n155 = Concatenate Strings(w49, w45, w48, w45, w44) -> (w47:string)
        n156 = Enqueue Element(queue=w61, element=w47) -> ()  [unwired: 2 in, 3 out]
        "Loop count" <- w65
      }
      n157 = node-c288(w26) -> ()  [unwired: 1 out]
      n158 = while {
        stop <- FALSE stop-if-true
        n159 = node-c288() -> (w451:T1)  [unwired: 4 in]
        n160 = Create Network Stream Reader Endpoint(7:10 ("reader buffer size"), 9:T5 {"Message"="", "Message Data"=variant} ("Message Cluster"), 11:"/command/reader/FGGA" ("reader url")) -> (0:w456:errorcluster, 3:w457:refnum<k21>)  [unwired: 4 in]
        n161 = timed-loop "Host->Target Command Reader" {
          shift-right: [w467] -> w454
          shift-left: w456 -> [w470]
          shift-right: [w468] -> w453
          shift-left: w457 -> [w469]
          tunnel: [TRUE] -> _
          timing: w451 -> [_]
          timing-out: [_] -> w450
          stop <- w461 stop-if-true
          # "Receive Commands from Host VI"
          n162 = node-c288() -> ()  [unwired: 1 in, 1 out]
          n163 = shared-variable-read(w469, w470) -> (w468:refnum<k21>, w463:errorcluster, w465:bool, w466:T5)  [unwired: 1 in]
          n164 = Or(x=w465, y=w463) -> (x .or. y?=w464:bool)
          n165 = case shown="False" w464 {
            selector: w464 -> [_ w534]
            tunnel: w463 -> [w478 w535]
            tunnel: [w477 w535] -> w467
            tunnel: w466 -> [w475 _]
            tunnel: [w476 w534] -> w461
            frame False {
              n166 = Unbundle By Name(w475) -> ("Message"=w474:string, "Message Data"=w473:variant)
              n167 = case shown="\"FGGA_pump\"" w474 {
                tunnel: w478 -> [w480 w485 w490 w495 w500 w505 w510 w515 w520 w528 w533]
                tunnel: [w480 w481 w489 w494 w499 w504 w509 w514 w519 w527 w532] -> w477
                tunnel: w473 -> [_ w484 w488 w493 w498 w503 w508 w513 w518 w526 w531]
                tunnel: [TRUE _ _ _ _ _ _ _ _ _ _] -> w476
                frame "Stop", Default {
                }
                frame "Stop File Write" {
                  n168 = Variant To Data(error in=w485, type=FALSE, Variant=w484) -> (data=→"Stop File Write":bool, error out=w481:errorcluster)
                }
                frame "V1" {
                  n169 = Variant To Data(error in=w490, type=FALSE, Variant=w488) -> (data=w486:bool, error out=w489:errorcluster)
                  "V1" <- w486
                  n170 = shared-variable "NI-cRIO9022-019C2C95\\Mod6\\DO0"(w486) -> ()  [unwired: 1 in, 1 out]
                }
                frame "V2" {
                  n171 = Variant To Data(error in=w495, type=FALSE, Variant=w493) -> (data=w491:bool, error out=w494:errorcluster)
                  "V2" <- w491
                  n172 = shared-variable "NI-cRIO9022-019C2C95\\Mod6\\DO1"(w491) -> ()  [unwired: 1 in, 1 out]
                }
                frame "V3" {
                  n173 = Variant To Data(error in=w500, type=FALSE, Variant=w498) -> (data=w496:bool, error out=w499:errorcluster)
                  "V3" <- w496
                  n174 = shared-variable "NI-cRIO9022-019C2C95\\Mod6\\DO2"(w496) -> ()  [unwired: 1 in, 1 out]
                }
                frame "V4" {
                  n175 = Variant To Data(error in=w505, type=FALSE, Variant=w503) -> (data=w501:bool, error out=w504:errorcluster)
                  "V4" <- w501
                  n176 = shared-variable "NI-cRIO9022-019C2C95\\Mod6\\DO3"(w501) -> ()  [unwired: 1 in, 1 out]
                }
                frame "MFC_1" {
                  n177 = Variant To Data(error in=w510, type=0.0, Variant=w508) -> (data=w506:dbl, error out=w509:errorcluster)
                  n178 = local write "MFC_1 SLPM set value"(w506) -> ()
                }
                frame "FGGA_restart" {
                  n179 = Variant To Data(error in=w515, type=FALSE, Variant=w513) -> (data=→"FGGA restart":bool, error out=w514:errorcluster)
                }
                frame "UDP Time Offset" {
                  n180 = Variant To Data(error in=w520, type=0, Variant=w518) -> (data=→"UDP Time Stamp Offset":i32, error out=w519:errorcluster)
                }
                frame "FGGA_pump" {
                  n181 = Variant To Data(error in=w528, type=FALSE, Variant=w526) -> (data=w523:bool, error out=w527:errorcluster)
                  "FGGA Pump" <- w523
                  n182 = Select(t=1.4 ("f"), s=w523, f=0.0 ("t")) -> (s? t:f=w524:dbl)
                  n183 = shared-variable "NI-cRIO9022-019C2C95\\Mod5\\AO0"(w524) -> ()  [unwired: 1 in, 1 out]
                }
                frame "Flight Number" {
                  n184 = Variant To Data(error in=w533, type="", Variant=w531) -> (data=→"Flight Number":string, error out=w532:errorcluster)
                }
              }
            }
            frame True {
            }
          }
          n185 = node-c288() -> ()  [unwired: 1 in, 1 out]
        }
        n186 = node-c288(w450) -> ()  [unwired: 1 out]
        n187 = Destroy Stream Endpoint(8:w454, 11:w453) -> (0:→"error out 2":errorcluster)
      }
      n188 = while {
        stop <- FALSE stop-if-true
        # "Emergency shutdown on the valves when connection to the client drops"
        n189 = shared-variable ".\\Global Shared Variables.lvlib\\Disconnect_WatchDog"() -> (w445:bool)  [unwired: 1 in, 1 out]
        n190 = Wait (ms)(milliseconds to wait=u32 1000) -> ()  [unwired: 1 out]
        n191 = case shown="True" w445 {
          frame False {
          }
          frame True {
            w449 = FALSE
            n192 = shared-variable "NI-cRIO9022-019C2C95\\Mod6\\DO1"(w449) -> ()  [unwired: 1 in, 1 out]
            n193 = shared-variable "NI-cRIO9022-019C2C95\\Mod6\\DO3"(w449) -> ()  [unwired: 1 in, 1 out]
            n194 = shared-variable "NI-cRIO9022-019C2C95\\Mod6\\DO0"(w449) -> ()  [unwired: 1 in, 1 out]
            n195 = shared-variable "NI-cRIO9022-019C2C95\\Mod6\\DO2"(w449) -> ()  [unwired: 1 in, 1 out]
            n196 = local write "MFC_1 SLPM set value"(0.0 ("MFC_1 SLPM set value")) -> ()
          }
        }
      }
      n197 = while {
        tunnel: w37 -> [w174]
        tunnel: w36 -> [w173]
        stop <- w175 stop-if-true
        # "Must Delay to avoid 100% CPU"
        # "Broadcast FGGA UDP Data"
        n198 = call-poly <vilib>:"UDP Multicast Open.vi"("time-to-live (1)"=u16 5, "port"=u16 10000) -> ("error out"=w182:errorcluster, "connection ID"=w183:refnum<k16>)  [unwired: 8 in]
        n199 = node-c288() -> (w185:T1)  [unwired: 4 in]
        n200 = timed-loop {
          tunnel: w183 -> [w206]
          tunnel: w182 -> [w205]
          timing: w185 -> [_]
          timing-out: [_] -> w184
          shift-right: [w194] -> _
          shift-left: FALSE -> [w197]
          tunnel: [w193] -> w177
          tunnel: [w191] -> w176
          tunnel: [w189] -> w175
          tunnel: w174 -> [w187]
          tunnel: w173 -> [w186]
          stop <- w190 stop-if-true
          # "UDP Broadcast loop"
          n201 = node-c288() -> ()  [unwired: 1 in, 1 out]
          n202 = local read "Flight Number"() -> (w188:string)
          n203 = feedback-in #2(w188) -> ()
          n204 = feedback #2() -> (w199:string)  [unwired: 1 in]
          n205 = Not Equal?(x=w188, y=w199) -> (x != y?=w198:bool)
          n206 = String To IP(1:"239.1.4.6" ("name")) -> (0:w203:u32)
          n207 = flat-sequence {
            tunnel: w203 -> [w213]
            tunnel: w205 -> [w214]
            tunnel: w206 -> [w215]
            tunnel: [w215] -> w202
            tunnel: [w214] -> w201
            tunnel: [w213] -> w200
            tunnel: w198 -> [w212]
            tunnel: u16 50001 ("port or service name") -> [w226]
            tunnel: w202 -> [w225]
            tunnel: w201 -> [w224]
            tunnel: w200 -> [w223]
            tunnel: [w222] -> w193
            tunnel: [w221] -> w191
            tunnel: w187 -> [w219]
            tunnel: w186 -> [w218]
            frame #0 {
              n208 = feedback #3(u32 0) -> (w209:u32)
              n209 = case shown="False" w212 {
                tunnel: w209 -> [w216 _]
                tunnel: [w216 u32 0] -> w208
                frame False {
                }
                frame True {
                }
              }
              "UDP_Pack_num" <- w208
              n210 = Increment(x=w208) -> (x+1=w210:u32)
              n211 = feedback-in #3(w210) -> ()
            }
            frame #1 {
              n212 = Dequeue Element(queue=w219, error in (no error)=w218) -> (element=w220:string)  [unwired: 1 in, 3 out]
              n213 = UDP Write(address=w223, port or service name=w226, connection ID=w225, data in=w220, 8:w224) -> (error out=w221:errorcluster, 3:w222:refnum<k16>)  [unwired: 1 in]
            }
          }
          n214 = Select(t=FALSE, s=w197, f=TRUE) -> (s? t:f=w194:bool)
          "UDP_Out Status" <- w194
          n215 = local read "stop"() -> (w189:bool)
          n216 = node-c288() -> ()  [unwired: 1 in, 1 out]
          n217 = Unbundle(w191) -> ("status"=w192:bool)  [unwired: 2 out]
          n218 = Compound Arithmetic op=OR(w192, w189) -> (w190:bool)
        }
        n219 = node-c288(w184) -> ()  [unwired: 1 out]
        n220 = UDP Close(connection ID=w177, 8:w176) -> (error out=→"UDP_Out_Error Out":errorcluster)  [unwired: 1 out]
        n221 = Wait (ms)(milliseconds to wait=u32 1000) -> ()  [unwired: 1 out]
      }
      n222 = while {
        tunnel: w33 -> [w132]
        tunnel: w32 -> [w131]
        stop <- w135 stop-if-true
        # "Must Delay to avoid 100% CPU"
        # "TCP Loop writing to FISH Tank"
        n223 = TCP Open Connection(address="192.168.101.110", remote port or service name=u16 3502) -> (connection ID=w138:refnum<k5>, error out=w133:errorcluster)  [unwired: 3 in]
        n224 = case shown="No Error" w133 {
          selector: w133 -> [w143 w170]
          tunnel: w138 -> [w148 w171]
          tunnel: [w147 w171] -> w137
          tunnel: [w146 w170] -> w136
          tunnel: [w145 w169] -> w135
          tunnel: w132 -> [w142 _]
          tunnel: w131 -> [w141 _]
          frame No Error {
            n225 = node-c288() -> (w150:T1)  [unwired: 4 in]
            n226 = timed-loop {
              tunnel: w148 -> [w164]
              tunnel: w143 -> [w163]
              tunnel: [w162] -> w147
              tunnel: [w161] -> w146
              tunnel: [w153] -> w145
              shift-right: [w155] -> _
              shift-left: FALSE -> [w158]
              timing: w150 -> [_]
              timing-out: [_] -> w149
              tunnel: w142 -> [w152]
              tunnel: w141 -> [w151]
              stop <- w159 stop-if-true
              n227 = node-c288() -> ()  [unwired: 1 in, 1 out]
              n228 = Dequeue Element(queue=w152, error in (no error)=w151) -> (element=w154:string)  [unwired: 1 in, 3 out]
              n229 = Select(t=FALSE, s=w158, f=TRUE) -> (s? t:f=w155:bool)
              "TCP packet\nSend To FISH" <- w155
              n230 = TCP Write(connection ID=w164, data in=w154, error in (no error)=w163) -> (connection ID out=w162:refnum<k5>, error out=w161:errorcluster)  [unwired: 1 in, 1 out]
              n231 = local read "stop"() -> (w153:bool)
              n232 = Unbundle(w161) -> ("status"=w160:bool)  [unwired: 2 out]
              n233 = node-c288() -> ()  [unwired: 1 in, 1 out]
              n234 = Compound Arithmetic op=OR(w160, w153) -> (w159:bool)
            }
            n235 = node-c288(w149) -> ()  [unwired: 1 out]
          }
          frame Error {
            n236 = local read "stop"() -> (w169:bool)
          }
        }
        n237 = TCP Close Connection(connection ID=w137, error in (no error)=w136) -> (error out=→"FISH TCP Error Out":errorcluster)  [unwired: 1 in, 1 out]
        n238 = Wait (ms)(milliseconds to wait=u32 1000) -> ()  [unwired: 1 out]
      }
      n239 = while {
        tunnel: w35 -> [w405]
        tunnel: w34 -> [w404]
        stop <- w408 stop-if-true
        # "Must Delay to avoid 100% CPU"
        # "TCP Loop writing to SEPTIC Tank"
        n240 = TCP Open Connection(address="192.168.101.108", remote port or service name=u16 3502) -> (connection ID=w411:refnum<k5>, error out=w406:errorcluster)  [unwired: 3 in]
        n241 = case shown="No Error" w406 {
          selector: w406 -> [w416 w443]
          tunnel: w411 -> [w421 w444]
          tunnel: [w420 w444] -> w410
          tunnel: [w419 w443] -> w409
          tunnel: [w418 w442] -> w408
          tunnel: w405 -> [w415 _]
          tunnel: w404 -> [w414 _]
          frame No Error {
            n242 = node-c288() -> (w423:T1)  [unwired: 4 in]
            n243 = timed-loop {
              tunnel: w421 -> [w437]
              tunnel: w416 -> [w436]
              tunnel: [w435] -> w420
              tunnel: [w434] -> w419
              tunnel: [w426] -> w418
              shift-right: [w428] -> _
              shift-left: FALSE -> [w431]
              timing: w423 -> [_]
              timing-out: [_] -> w422
              tunnel: w415 -> [w425]
              tunnel: w414 -> [w424]
              stop <- w432 stop-if-true
              n244 = node-c288() -> ()  [unwired: 1 in, 1 out]
              n245 = Dequeue Element(queue=w425, error in (no error)=w424) -> (element=w427:string)  [unwired: 1 in, 3 out]
              n246 = Select(t=FALSE, s=w431, f=TRUE) -> (s? t:f=w428:bool)
              "TCP packet\nSend To SEPTIC" <- w428
              n247 = TCP Write(connection ID=w437, data in=w427, error in (no error)=w436) -> (connection ID out=w435:refnum<k5>, error out=w434:errorcluster)  [unwired: 1 in, 1 out]
              n248 = local read "stop"() -> (w426:bool)
              n249 = Unbundle(w434) -> ("status"=w433:bool)  [unwired: 2 out]
              n250 = node-c288() -> ()  [unwired: 1 in, 1 out]
              n251 = Compound Arithmetic op=OR(w433, w426) -> (w432:bool)
            }
            n252 = node-c288(w422) -> ()  [unwired: 1 out]
          }
          frame Error {
            n253 = local read "stop"() -> (w442:bool)
          }
        }
        n254 = TCP Close Connection(connection ID=w410, error in (no error)=w409) -> (error out=→"SEPTIC TCP Error Out":errorcluster)  [unwired: 1 in, 1 out]
        n255 = Wait (ms)(milliseconds to wait=u32 1000) -> ()  [unwired: 1 out]
      }
    }
    frame Error {
    }
  }
  n256 = VISA Close(VISA resource name=w17, error in (no error)=w18) -> (error out=→"Serial error out":errorcluster)
